vi "ShockTestImpedance_V2.vi"() -> ()   [LabVIEW 2021]
uses:
  <vilib>/express/express analysis/Spectral/Block/exnSpectralBlock spectral measurements RMS poly.vi
  <vilib>/express/express analysis/Spectral/Block/exnSpectralBlock spectral measurements RMS DDT.vi
  <vilib>/express/express analysis/Spectral/XNode/ExpressSpectralMeasurementsBlockNode.xnode
panel:
  out "error out":errorcluster
  out "Waveform Graph":dynamicdata(graph)
  out "x > 0? 2":bool
  out "x > 0?":bool
  out "return count":u32
  out "VISA resource name out":refnum<visa-resource-name>
  out "current sample":string
  out "data":dynamicdata(graph)
  in  "error in (no error)":errorcluster
  in  "VISA resource name":refnum<visa-resource-name>
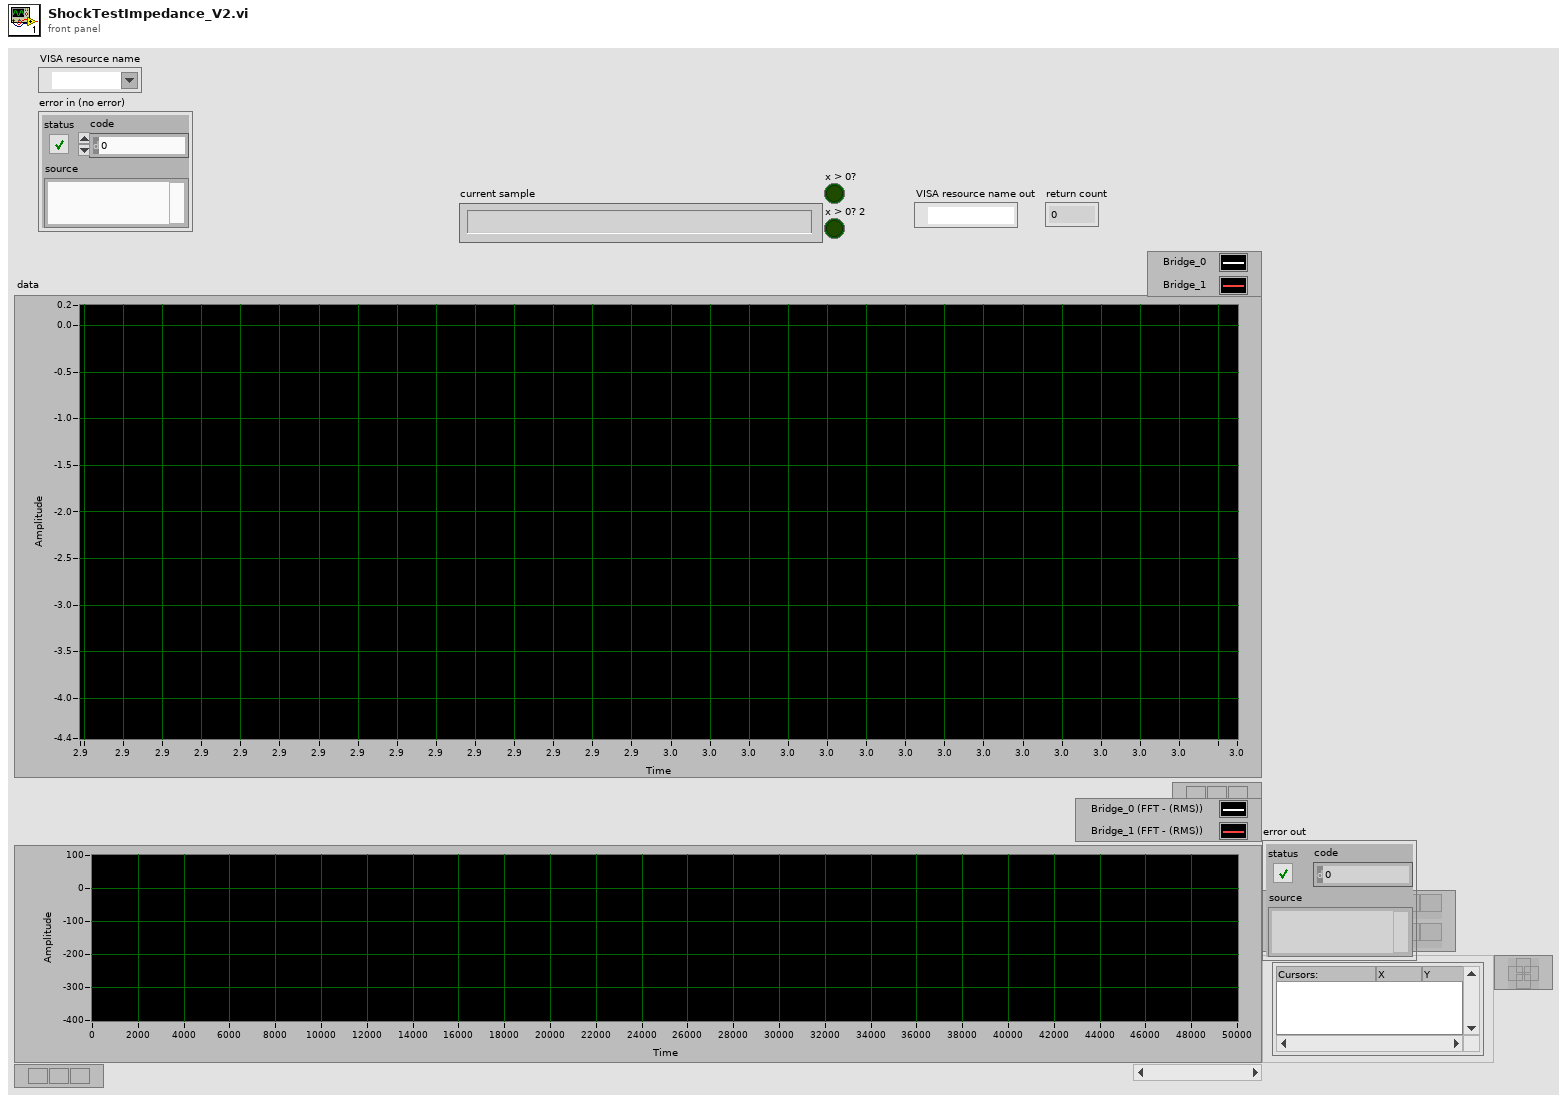
[diagram p1: front panel]
types:
  T1 = cluster{"averaging mode":u16, "weighting mode":u16, "number of averages":u32}
  T2 = cluster{"dB On (F)":bool, "unwrap phase (F)":bool, "convert to degree (F)":bool}
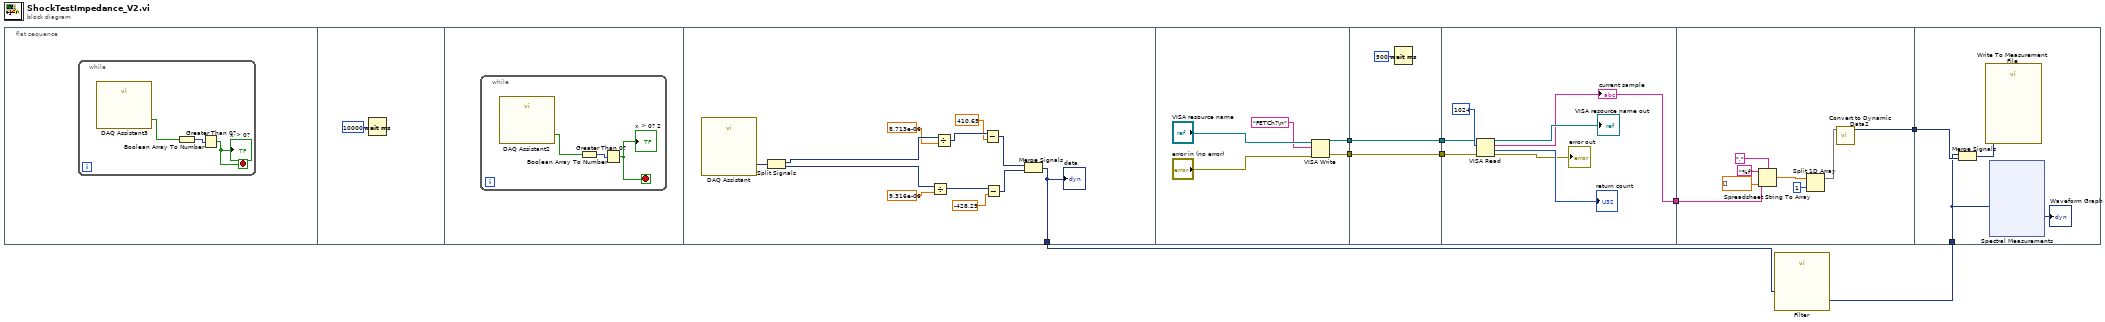
[diagram p0: block diagram]
diagram:
  n1 = flat-sequence {
    tunnel: [w16] -> w2
    tunnel: [w29] -> w8
    tunnel: [w28] -> w7
    tunnel: w8 -> [w35]
    tunnel: w7 -> [w34]
    tunnel: [w35] -> w6
    tunnel: [w34] -> w5
    tunnel: w6 -> [w38]
    tunnel: w5 -> [w39]
    tunnel: [w37] -> w4
    tunnel: w4 -> [w45]
    tunnel: [w43] -> w3
    tunnel: w3 -> [w53]
    tunnel: w1 -> [w52]
    frame #0 {
      n2 = while {
        stop <- w9 stop-if-true
        n3 = call "DAQ Assistant3"() -> ("data"=w11:bool[])  [unwired: 17 in, 2 out]
        n4 = Boolean Array To Number(Boolean array=w11) -> (number=w10:u32)
        n5 = Greater Than 0?(x=w10) -> (x > 0?=w9:bool)
        "x > 0?" <- w9
      }
    }
    frame #1 {
      n6 = Wait (ms)(milliseconds to wait=u32 10000) -> ()  [unwired: 1 out]
    }
    frame #2 {
      n7 = while {
        stop <- w13 stop-if-true
        n8 = call "DAQ Assistant2"() -> ("data"=w15:bool[])  [unwired: 17 in, 2 out]
        n9 = Boolean Array To Number(Boolean array=w15) -> (number=w14:u32)
        n10 = Greater Than 0?(x=w14) -> (x > 0?=w13:bool)
        "x > 0? 2" <- w13
      }
    }
    frame #3 {
      n11 = call "DAQ Assistant"() -> ("data"=w21:dynamicdata)  [unwired: 17 in, 2 out]
      n12 = Split Signals(w21) -> (w26:dynamicdata, w27:dynamicdata)  [unwired: 2 in]
      n13 = Divide(x=w27, y=9.316e-06) -> (x/y=w25:dynamicdata)
      n14 = Divide(x=w26, y=8.713e-06) -> (x/y=w24:dynamicdata)
      n15 = Subtract(x=w24, y=410.65) -> (x-y=w22:dynamicdata)
      n16 = Subtract(x=w25, y=-428.25) -> (x-y=w23:dynamicdata)
      n17 = Merge Signals(w22, w23) -> (w16:dynamicdata)
      "data" <- w16
    }
    frame #4 {
      n18 = VISA Write(VISA resource name="VISA resource name", write buffer="FETCh?\n" ("Command"), error in (no error)="error in (no error)") -> (VISA resource name out=w28:refnum<visa-resource-name>, error out=w29:errorcluster)  [unwired: 1 out]
    }
    frame #5 {
      n19 = Wait (ms)(milliseconds to wait=u32 500 ("delay before read (ms)")) -> ()  [unwired: 1 out]
    }
    frame #6 {
      n20 = VISA Read(VISA resource name=w39, byte count=u32 1024, error in (no error)=w38) -> (VISA resource name out=→"VISA resource name out":refnum<visa-resource-name>, read buffer=w37:string, return count=→"return count":u32, error out=→"error out":errorcluster)
      "current sample" <- w37
    }
    frame #7 {
      n21 = Spreadsheet String To Array(delimiter (Tab)=",", format string="%f", spreadsheet string=w45, array type (2D Dbl)=dbl[] []) -> (array=w49:dbl[])
      n22 = Split 1D Array(array=w49, index=1) -> (first subarray=w50:dbl[])  [unwired: 1 out]
      n23 = call "Convert to Dynamic Data2"("Array"=w50) -> ("Dynamic Data Type"=w43:dynamicdata)  [unwired: 3 in]
    }
    frame #8 {
      n24 = Merge Signals(w52, w53) -> (w54:dynamicdata)
      n25 = call "Write To Measurement File"("Signals"=w54) -> ()  [unwired: 16 in, 3 out]
      n26 = xnode "Spectral Measurements"("Signals"=w52) -> ("FFT - (RMS)"=→"Waveform Graph":dynamicdata)  [unwired: 1 in, 2 out]
    }
  }
  n27 = call "Filter"("Signal"=w2) -> ("Filtered Signal"=w1:dynamicdata)  [unwired: 9 in, 1 out]
